vi "Set Status Error Channel Data References.vi"(8 "error in":errorcluster, 10 "custom device ref in":T1 format="%.0x", 11 "Ballard ARINC-429 Rx Execution Unit in":refnum<class "Ballard ARINC-429 Rx Execution Unit.lvclass">) -> (0 "error out":errorcluster, 3 "Ballard ARINC-429 Rx Execution Unit out":refnum<class "Ballard ARINC-429 Rx Execution Unit.lvclass">)   [LabVIEW 2020]
uses:
  Engine/Implementation/Ballard ARINC-429 Rx Execution Unit/Ballard ARINC-429 Rx Execution Unit.lvclass
  <vilib>/NI VeriStand/Custom Device API/Custom Device Item Ref.ctl
  <vilib>/NI VeriStand/Custom Device API/Data Reference.ctl
  <vilib>/NI VeriStand/Custom Device API/Data Access Type.ctl
  Engine/Implementation/Ballard ARINC-429 Rx Execution Unit/Ballard ARINC-429 Rx Execution Unit.lvclass/Ballard ARINC-429 Rx Execution Unit.ctl
  Engine/Implementation/Ballard ARINC-429 Rx Execution Unit/Write Status Error Channel Data References.vi
  Scripting/Ballard ARINC 429 Scripting.lvlib
  <vilib>/NI VeriStand/Custom Device API/Custom Device API.lvlib
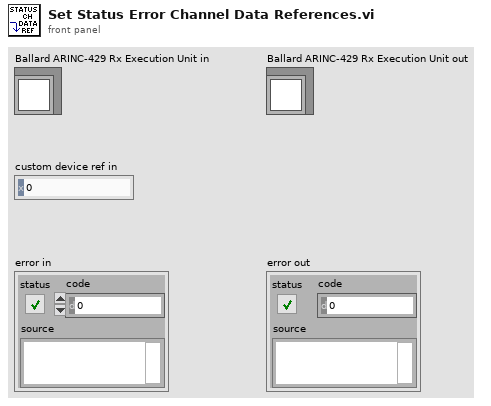
[diagram p1: front panel]
types:
  T1 = typedef "Custom Device API.lvlib/Custom Device Item Ref.ctl" = u64
  T2 = typedef "Custom Device API.lvlib/Data Access Type.ctl" = enum16{"Read", "Write"}
  T3 = typedef "Custom Device API.lvlib/Data Reference.ctl" = i32
  T4 = cluster{"receiving":T3, "specific errors":cluster{"gap":T3, "parity":T3, "long word ":T3, "bit timing":T3, "timeout":T3}}
  T5 = cluster{"gap":T1, "parity":T1, "long word":T1, "bit timing":T1, "timeout":T1}
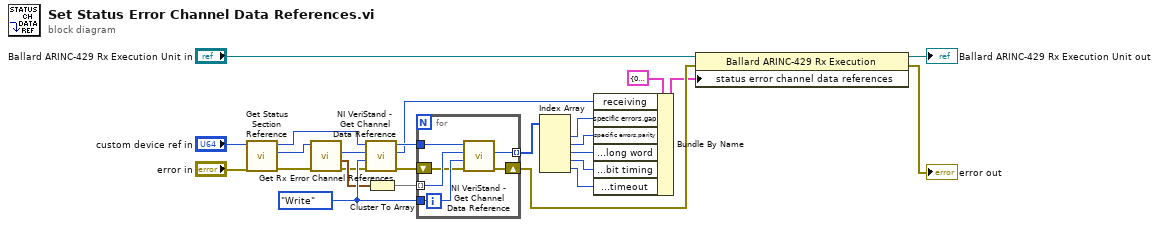
[diagram p0: block diagram]
diagram:
  w18 = Data_Access_Type."Write" ("Access")
  n1 = call "Get Status Section Reference.vi"("error in"="error in", "Ballard ARINC 429 ref"="custom device ref in") -> ("error out"=w23:errorcluster, "status section reference"=w24:T1, "Ballard ARINC 429 ref out"=w1:T1)  [unwired: 7 in]
  n2 = call "Get Rx Error Channel References.vi"("error in"=w23, "status reference in"=w24) -> ("error out"=w15:errorcluster, "Rx specific error count references"=w16:T5, "Rx error count reference"=w19:T1)  [unwired: 6 in, 1 out]
  n3 = call <vilib>:"NI VeriStand - Get Channel Data Reference.vi"("error in (no error)"=w15, "Access"=w18, "Channel Ref in"=w19, "Device Ref in"=w1) -> ("error out"=w13:errorcluster, "Channel Data Reference"=w6:T3, "Device Ref out"=w17:T1)  [unwired: 5 in]
  n4 = Cluster To Array(cluster=w16) -> (array=w14:T1[])
  n5 = for {
    tunnel: w18 -> [w31]
    tunnel: w17 -> [w30]
    tunnel: w14 -> [w29] mode=indexing
    tunnel: [w27] -> w12 mode=indexing
    shift-right: [w26] -> w3
    shift-left: w13 -> [w28]
    n6 = call <vilib>:"NI VeriStand - Get Channel Data Reference.vi"("error in (no error)"=w28, "Access"=w31, "Channel Ref in"=w29, "Device Ref in"=w30) -> ("error out"=w26:errorcluster, "Channel Data Reference"=w27:T3)  [unwired: 5 in, 1 out]
  }
  n7 = Index Array(array=w12) -> (element #1=w11:T3, element #2=w10:T3, element #3=w9:T3, element #4=w8:T3, element #5=w7:T3)  [unwired: 5 in]
  n8 = Bundle By Name(cluster=T4 {"receiving"=0, "specific errors"={"gap"=0, "parity"=0, "long word "=0, "bit timing"=0, "timeout"=0}} ("status error channel data references"), "receiving"=w6, "specific errors.gap"=w11, "specific errors.parity"=w10, "specific errors.long word"=w9, "specific errors.bit timing"=w8, "specific errors.timeout"=w7) -> (w2:T4)
  n9 = property class="Ballard ARINC-429 Rx Execution "(reference="Ballard ARINC-429 Rx Execution Unit in", error in=w3, "status error channel data references"=w2) -> (reference out=→"Ballard ARINC-429 Rx Execution Unit out":refnum<class "Ballard ARINC-429 Rx Execution Unit.lvclass">, error out=→"error out":errorcluster)
